vi "Get-path-string-table.vi"(8 "error in (no error)":errorcluster, 11 "Reference in":T1) -> (0 "error out":errorcluster, 2 "String table":string[][](array[string]), 3 "Reference out":T1)   [LabVIEW 2013, in "MaterialCharacterization.lvlib" / "MC-ScanParser.lvclass"]
uses:
  MC-ScanParser.lvclass
  Object-reference.ctl
  MC-ScanParser.lvclass/MC-ScanParser.ctl
  Read Path.vi
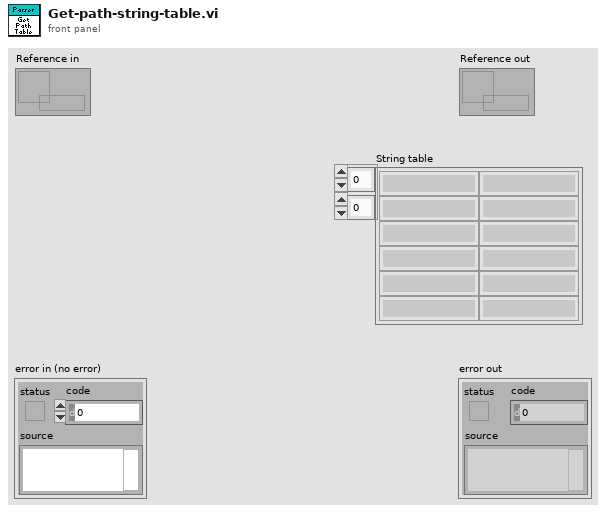
[diagram p1: front panel]
types:
  T1 = typedef "MaterialCharacterization.lvlib/MC-ScanParser.lvclass/Object-reference.ctl" = refnum<data-value>
  T2 = typedef "HardwareCharacterization.lvlib/HC-ScanParser.lvclass/Point-buffer.ctl" = cluster{"Start time [µs]":i64, "End time [µs]":i64, "X [mm]":dbl, "Y [mm]":dbl, "Type":T3, "Speed [mm/µs]":dbl, "Direction [rad]":dbl, "X [bit]":i16, "Y [bit]":i16, "Speed [bit/µs]":dbl, "Power [W]":dbl, "Power [bit]":u8, "JumpDelay":i64, "MarkDelay":i64, "PolyDelay":i64, "LaserOnDelay":i64, "LaserOffDelay":i64, "LaserPowerDelay":i64, "LaserEnableDelay":i64, "Xraw [mm]":dbl, "Yraw [mm]":dbl}
  T3 = typedef "HardwareCharacterization.lvlib/Element-XML.lvclass/Elements.ctl" = enum16{"BeginJob", "WriteDigital", "WriteAnalog", "Set", "ApplicationEvent", "JumpAbs", "MarkAbs", "JumpRel", "MarkRel", "LongDelay", "EndJob"}
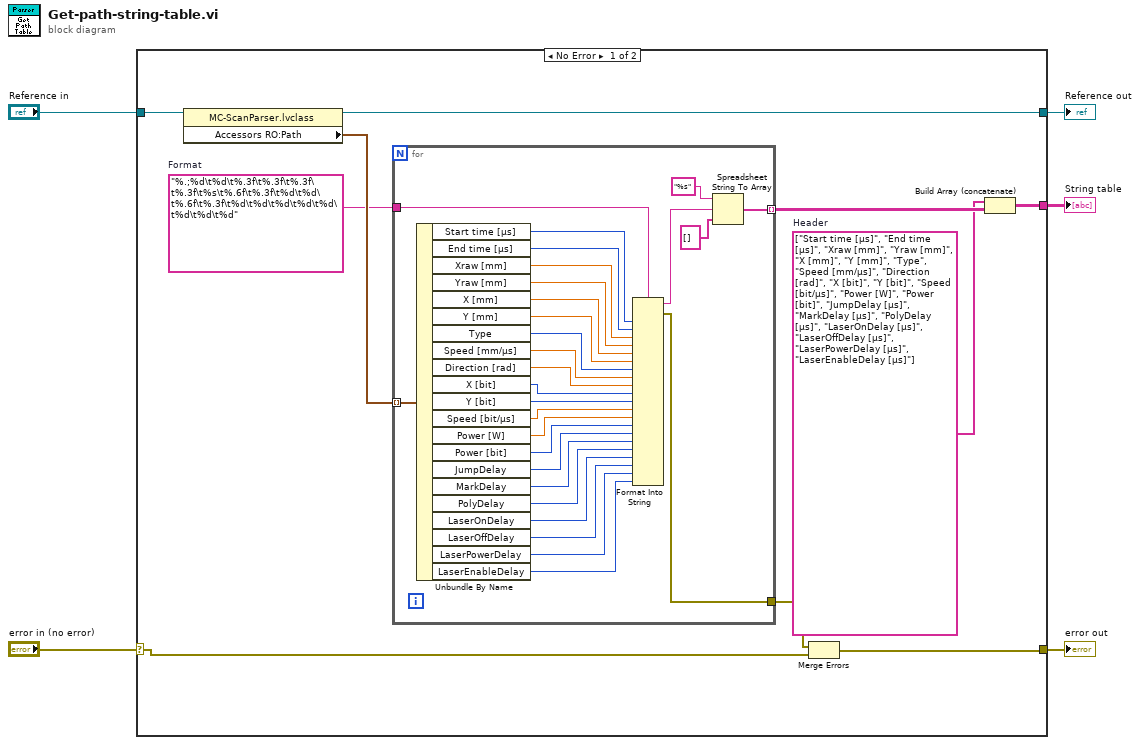
[diagram p0: block diagram]
diagram:
  n1 = case shown="No Error" "error in (no error)" {
    selector: "error in (no error)" -> [w6 w44]
    tunnel: [w8 w44] -> w4
    tunnel: [w14 w45] -> w2
    tunnel: "Reference in" -> [w15 w45]
    tunnel: [w9 _] -> w1
    frame No Error {
      w10 = string[] ["Start time [µs]", "End time [µs]", "Xraw [mm]", "Yraw [mm]", "X [mm]", "Y [mm]", "Type", "Speed [mm/µs]", "Direction [rad]", "X [bit]", "Y [bit]", "Speed [bit/µs]", "Power [W]", "Power [bit]", "JumpDelay [µs]", "MarkDelay [µs]", "PolyDelay [µs]", "LaserOnDelay [µs]", "LaserOffDelay [µs]", "LaserPowerDelay [µs]", "LaserEnableDelay [µs]"]  # Header
      w12 = "%.;%d\t%d\t%.3f\t%.3f\t%.3f\t%.3f\t%s\t%.6f\t%.3f\t%d\t%d\t%.6f\t%.3f\t%d\t%d\t%d\t%d\t%d\t%d\t%d\t%d"  # Format
      n2 = property class="MC-ScanParser.lvclass"(reference=w15) -> (reference out=w14:T1, "Accessors RO:Path"=w13:T2[])  [unwired: 1 in, 1 out]
      n3 = for {
        tunnel: w13 -> [w43] mode=indexing
        tunnel: w12 -> [w40]
        tunnel: [w18] -> w11 mode=indexing
        tunnel: [w17] -> w7
        n4 = Unbundle By Name(w43) -> ("Start time [µs]"=w42:i64, "End time [µs]"=w41:i64, "Xraw [mm]"=w39:dbl, "Yraw [mm]"=w38:dbl, "X [mm]"=w37:dbl, "Y [mm]"=w36:dbl, "Type"=w35:T3, "Speed [mm/µs]"=w34:dbl, "Direction [rad]"=w33:dbl, "X [bit]"=w32:i16, "Y [bit]"=w31:i16, "Speed [bit/µs]"=w30:dbl, "Power [W]"=w29:dbl, "Power [bit]"=w28:u8, "JumpDelay"=w27:i64, "MarkDelay"=w26:i64, "PolyDelay"=w25:i64, "LaserOnDelay"=w24:i64, "LaserOffDelay"=w23:i64, "LaserPowerDelay"=w22:i64, "LaserEnableDelay"=w21:i64)
        n5 = Format Into String(format string=w40, w42, w41, w39, w38, w37, w36, w35, w34, w33, w32, w31, w30, w29, w28, w27, w26, w25, w24, w23, w22, w21) -> (resulting string=w20:string, error out=w17:errorcluster)  [unwired: 2 in]
        n6 = Spreadsheet String To Array(format string="%s", spreadsheet string=w20, array type (2D Dbl)=string[] []) -> (array=w18:string[])  [unwired: 1 in]
      }
      n7 = Merge Errors(w7, w6) -> (w8:errorcluster)
      n8 = Build Array (concatenate)(w10, w11) -> (w9:string[][])
    }
    frame Error {
    }
  }
  "error out" <- w4
  "Reference out" <- w2
  "String table" <- w1
